vi "3D Single Mouse Movie.vi"() -> ()   [LabVIEW 2011]
uses:
  <vilib>/Native 3D Graph/xcontrol/3DPC_SurfacePlot.xctl
  <vilib>/Analysis/3filter.llb/Filter Passband Type.ctl
  <vilib>/Utility/file.llb/Write To Spreadsheet File (string).vi
  <vilib>/Analysis/1siggen.llb/Ramp Pattern by Samples.vi
  <vilib>/measure/mascope.llb/Transition Measurements 1 chan.vi
  <vilib>/Utility/file.llb/Write To Spreadsheet File (DBL).vi
  <vilib>/gmath/statdist.llb/Wilcoxon Signed-Rank Test (mean).vi
  <vilib>/vision/NI_Vision_Development_Module.lvlib
  <vilib>/Analysis/NI_AALBase.lvlib
  <vilib>/ptbypt/NI_PtbyPt.lvlib
  <vilib>/gmath/NI_Gmath.lvlib
  <vilib>/Analysis/NI_AALPro.lvlib
  <vilib>/Analysis/NI_AAL_Geometry.lvlib
  <vilib>/measure/NI_MAPro.lvlib
panel:
  out "Particle Measurements (Pixels)":dbl[][](array[numeric]) format="%.2f"
  in  "Selection Values":T2(array[cluster]) {"Measurement Parameter" items=["Center of Mass X", "Center of Mass Y", "First Pixel X", "First Pixel Y", "Bounding Rect Left", "Bounding Rect Top", "Bounding Rect Right", "Bounding Rect Bottom", "Max Feret Diameter Start X", "Max Feret Diameter Start Y", "Max Feret Diameter End X", "Max Feret Diameter End Y", "Max Horiz. Segment Length Left", "Max Horiz. Segment Length Right", "Max Horiz. Segment Length Row", "-", "Bounding Rect Width", "Bounding Rect Height", "Bounding Rect Diagonal", "Perimeter", "Convex Hull Perimeter", "Holes' Perimeter", "Max Feret Diameter", "Equivalent Ellipse Major Axis", "Equivalent Ellipse Minor Axis", "Equivalent Ellipse Minor Axis (Feret)", "Equivalent Rect Long Side", "Equivalent Rect Short Side", "Equivalent Rect Diagonal", "Equivalent Rect Short Side (Feret)", "Average Horiz. Segment Length", "Average Vert. Segment Length", "Hydraulic Radius", "Waddel Disk Diameter", "-", "Area", "Holes' Area", "Particle & Holes' Area", "Convex Hull Area", "Image Area", "-", "Number of Holes", "Number of Horiz. Segments", "Number of Vert. Segments", "-", "Orientation", "Max Feret Diameter Orientation", "-", "% Area/Image Area", "% Area/(Particle & Holes' Area)", "Ratio of Equivalent Ellipse Axes", "Ratio of Equivalent Rect Sides", "-", "Elongation Factor", "Compactness Factor", "Heywood Circularity Factor", "Type Factor", "-", "Sum X", "Sum Y", "Sum XX", "Sum XY", "Sum YY", "Sum XXX", "Sum XXY", "Sum XYY", "Sum YYY", "-", "Moment of Inertia XX", "Moment of Inertia XY", "Moment of Inertia YY", "Moment of Inertia XXX", "Moment of Inertia XXY", "Moment of Inertia XYY", "Moment of Inertia YYY", "Norm. Moment of Inertia XX", "Norm. Moment of Inertia XY", "Norm. Moment of Inertia YY", "Norm. Moment of Inertia XXX", "Norm. Moment of Inertia XXY", "Norm. Moment of Inertia XYY", "Norm. Moment of Inertia YYY", "Hu Moment 1", "Hu Moment 2", "Hu Moment 3", "Hu Moment 4", "Hu Moment 5", "Hu Moment 6", "Hu Moment 7"]; "Range Lower Value" format="%.2f"; "Range Upper Value" format="%.2f"}
  out "3D Graph":refnum<class "Base Datatype.lvclass">[](xcontrol)
  out "Spine Area v Max Height, 1 second history":T3(graph)
  in  "Image Folder":path=path "C:/Users/Behavior Room/Desktop/Recordings/Mouse 3"
  in  "Recording File":path=path "C:/Users/Behavior Room/Dropbox/Science/Datta lab/Kinect Mouse/Analysis/Blah.csv"
  in  "low cutoff freq: fl":dbl=0.125 format="%0.3f"
  out "Velocity":dbl(slide) scale=0.0..10.0
  in  "Flip?":bool
  in  "Butt Position":i32=10
  in  "threshold":dbl=100.0
  in  "Width of Band to \nCalculate Average Contour":i32=10
  out "Height":dbl(graph)
  out "Heat Map":T4(plugin-control)
  in  "Kernel Size":i32=11
  out "Right":bool
  out "Left":bool
  out "Is Significant":bool
  out "Half-Image Variance":T5(graph)
  out "Cross-Sectional Contour":cluster{"Y Max":i16[], "Ramp Pattern":dbl[]}(graph)
  out "Spine Contour":i16[][](graph) caption="X"
  in  "3D options":T6={"alpha"=15.0, "beta"=31.0, "border"=20, "background"=85, "plane"=2} {"beta" min=15 max=45 format="%.2f"; "alpha" min=15 max=45 format="%.2f"}
  in  "Direction (NW)":T7(ring)
  in  "Maximum height":i32=20
  in  "Size reduction":i32=1
  out "3D Experiment Area View":T4(plugin-control)
  out "Just Mouse":T4(plugin-control)
  out "Image #":i32
  out "Image":T4(plugin-control)
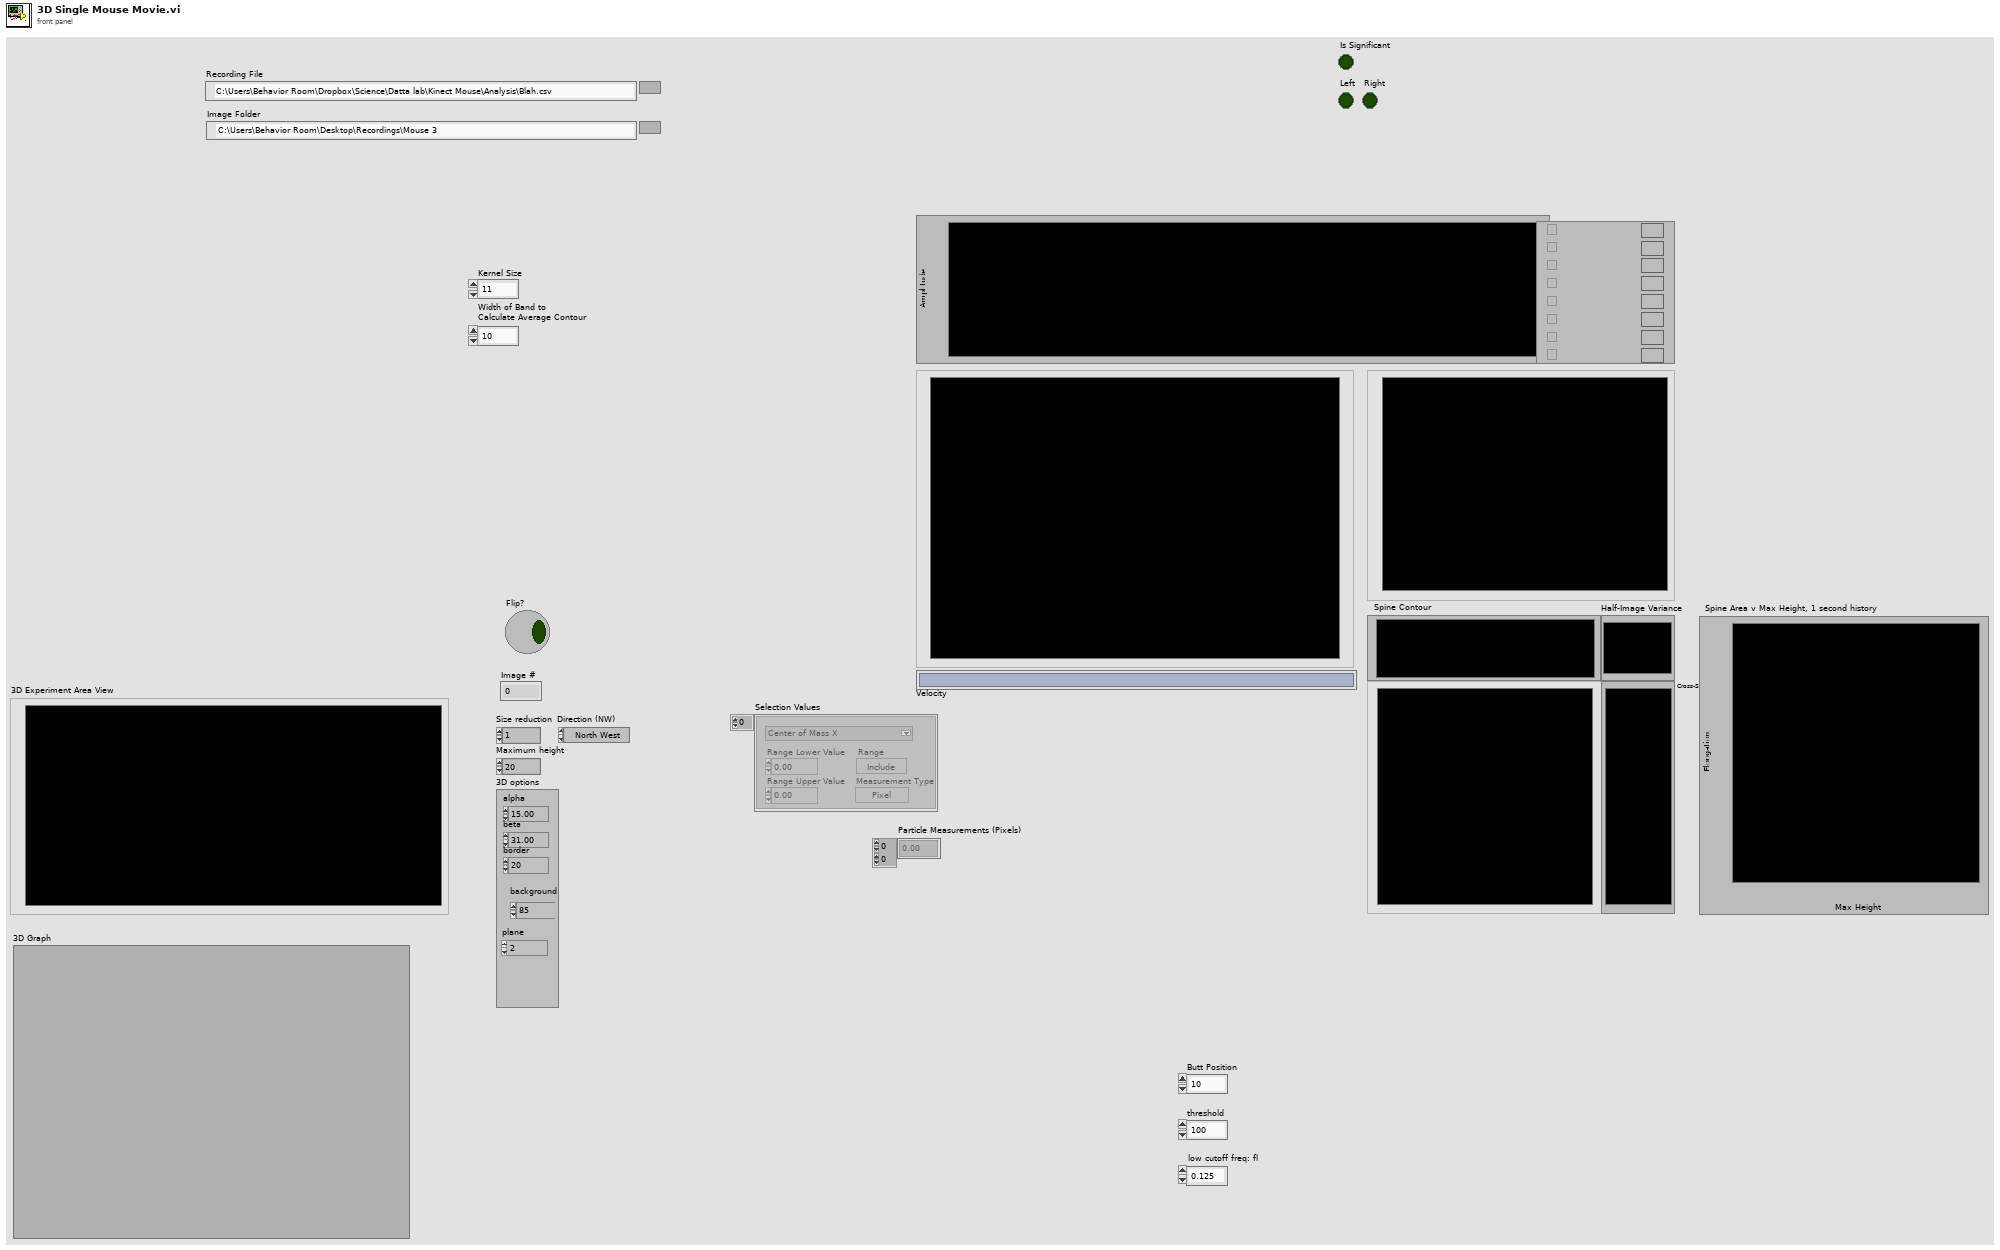
[diagram p1: front panel]
types:
  T1 = typedef "Particle Parameters" = i32
  T2 = cluster{"Measurement Parameter":T1, "Range Lower Value":dbl, "Range Upper Value":dbl, "Range":bool, "Measurement Type":bool}[]
  T3 = cluster{"Current Queue":dbl[], "Current Queue":dbl[]}
  T4 = typedef "IMAQ Image.ctl" = refnum<image>
  T5 = cluster{"standard deviation":dbl, "standard deviation":dbl}
  T6 = cluster{"alpha":sgl, "beta":sgl, "border":i32, "background":i32, "plane":i32}
  T7 = enum32{"North West", "South West", "South East", "North East"}
  T8 = typedef "Image Type" = u32
  T9 = typedef "NI_AALBase.lvlib/Filter Passband Type.ctl" = enum32{"Lowpass", "Highpass", "Bandpass", "Bandstop"}
  T10 = cluster{"Area":dbl, "Number of Holes":dbl, "Bounding Rect":cluster{"Left":dbl, "Top":dbl, "Right":dbl, "Bottom":dbl}, "Center of Mass":cluster{"X":dbl, "Y":dbl}, "Orientation":dbl, "Dimensions":cluster{"Width":dbl, "Height":dbl}}[]
  T11 = cluster{"high ref level":dbl, "mid ref level":dbl, "low ref level":dbl, "ref units":u16}
  T12 = cluster{"Area":dbl, "Number of Holes":dbl, "Bounding Rect":cluster{"Left":dbl, "Top":dbl, "Right":dbl, "Bottom":dbl}, "Center of Mass":cluster{"X":dbl, "Y":dbl}, "Orientation":dbl, "Dimensions":cluster{"Width":dbl, "Height":dbl}}
  T13 = cluster{"start time":dbl, "end time":dbl, "ref levels":cluster{"high ref level":dbl, "mid ref level":dbl, "low ref level":dbl, "ref units":u16}}
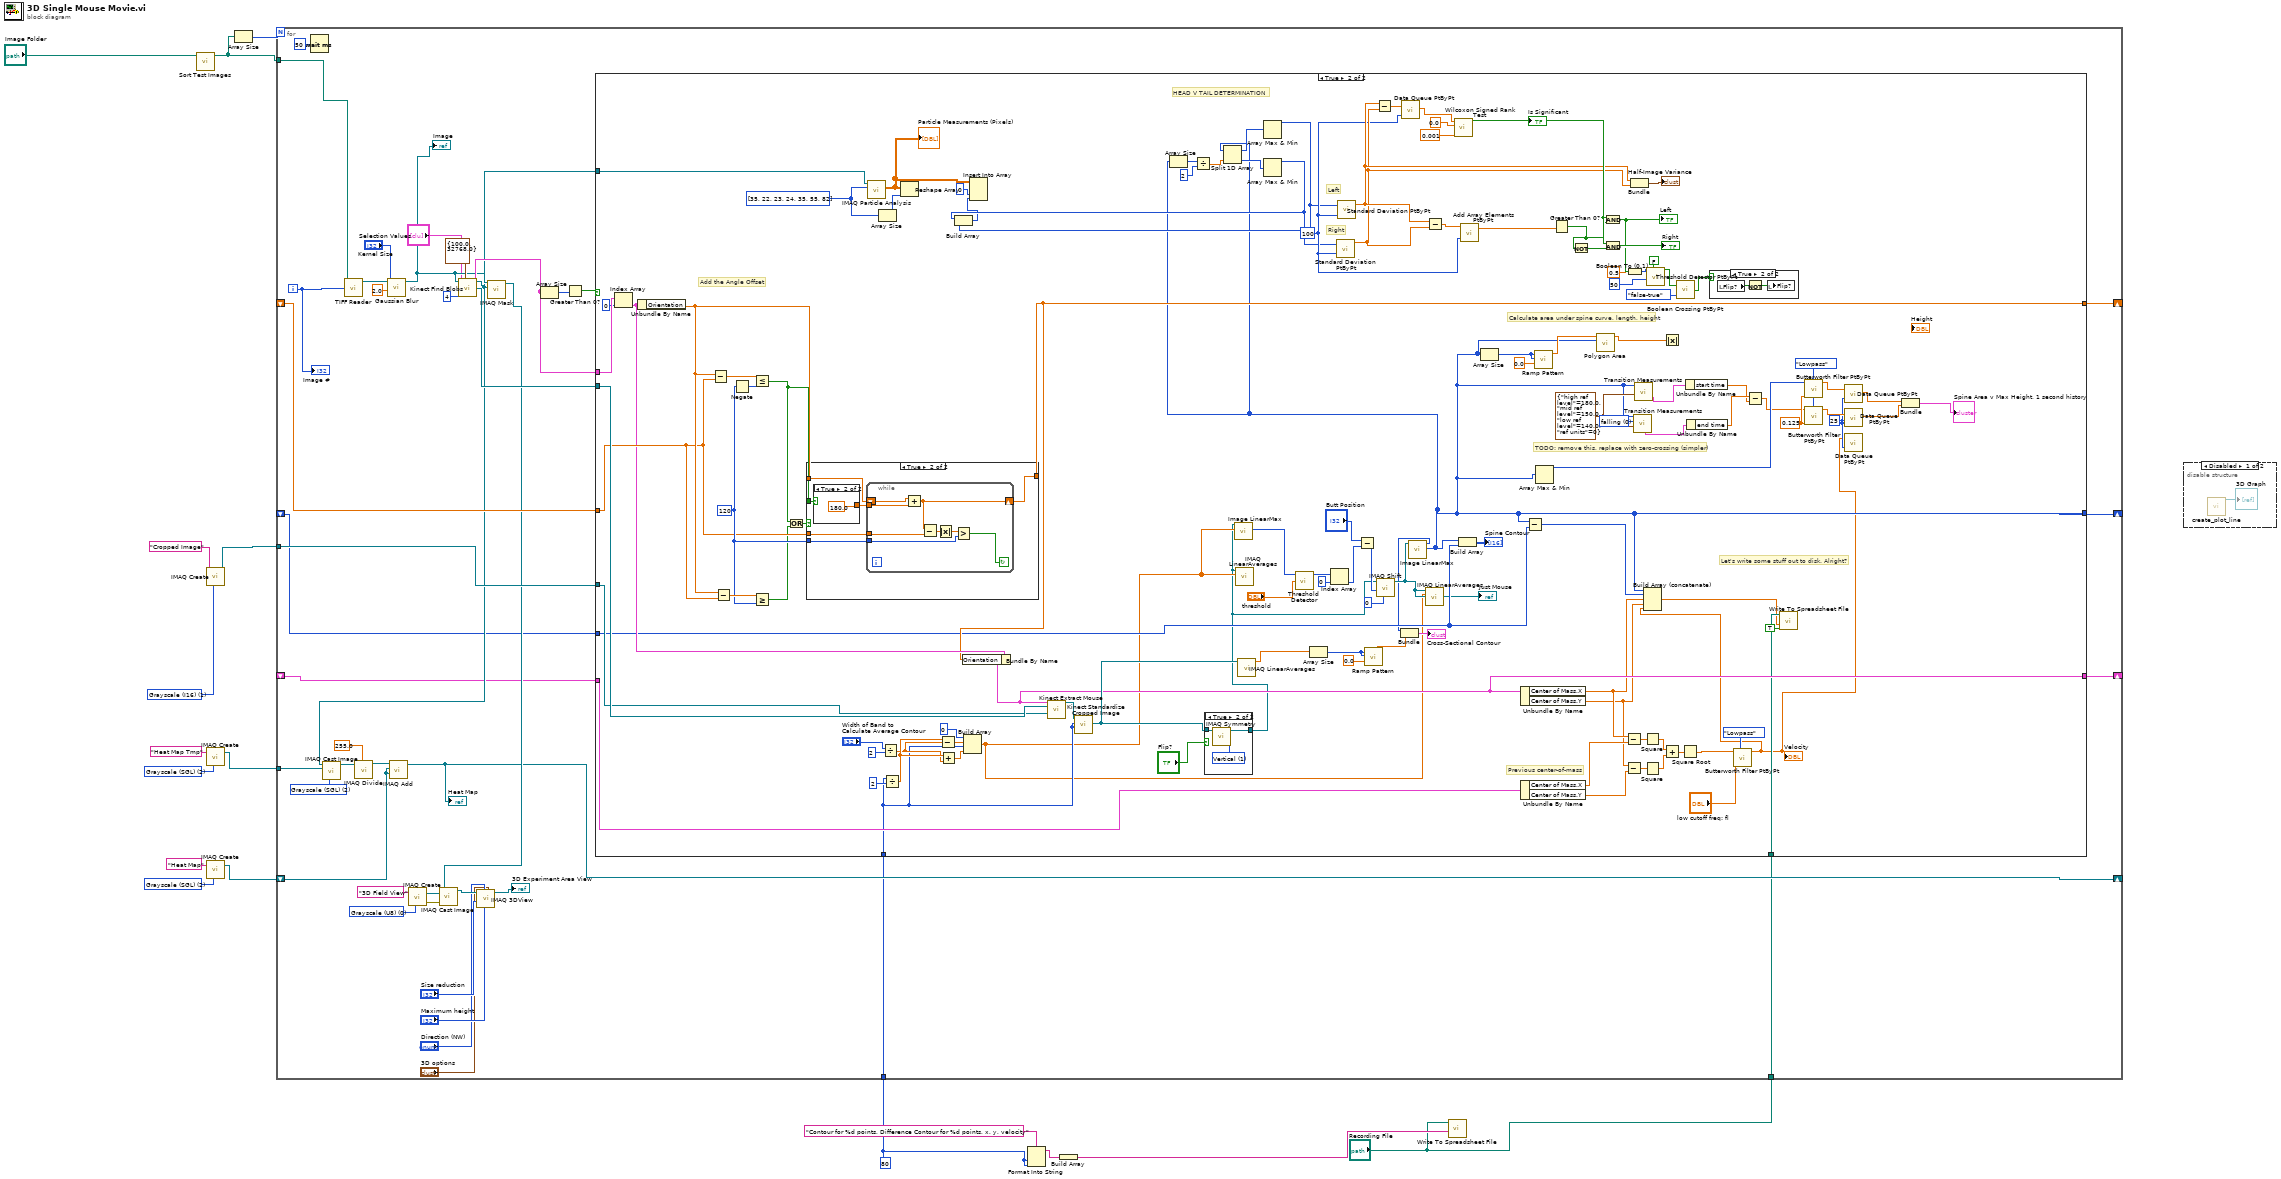
[diagram p0: block diagram]
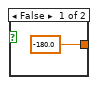
[diagram p6: hidden frame]
diagram:
  w4 = 80 ("Width")
  w7 = T8 2 items=["Grayscale (U8)", "Grayscale (I16)", "Grayscale (SGL)", "Complex (CSG)", "RGB (U32)", "HSL (U32)", "RGB (U64)", "Grayscale (U16)"] ("Image Type")
  w11 = T8 2 items=["Grayscale (U8)", "Grayscale (I16)", "Grayscale (SGL)", "Complex (CSG)", "RGB (U32)", "HSL (U32)", "RGB (U64)", "Grayscale (U16)"] ("Image Type")
  w14 = T8 1 items=["Grayscale (U8)", "Grayscale (I16)", "Grayscale (SGL)", "Complex (CSG)", "RGB (U32)", "HSL (U32)", "RGB (U64)", "Grayscale (U16)"] ("Image Type")
  n1 = call "Sort Test Images.vi"("path"="Image Folder") -> ("Array"=w16:path[])  [unwired: 10 in]
  n2 = call "IMAQ Create"("Image Name"="Cropped Image", "Image Type"=w14) -> ("New Image"=w13:T4)  [unwired: 3 in, 1 out]
  n3 = call "IMAQ Create"("Image Name"="Heat Map Tmp", "Image Type"=w7) -> ("New Image"=w6:T4)  [unwired: 3 in, 1 out]
  n4 = call "IMAQ Create"("Image Name"="Heat Map", "Image Type"=w11) -> ("New Image"=w9:T4)  [unwired: 3 in, 1 out]
  n5 = Array Size(array=w16) -> (size(s)=w17:i32)
  n6 = for {
    N: w17 -> [_]
    tunnel: w16 -> [w59]
    tunnel: w13 -> [w53]
    shift-right: [w51] -> _
    shift-left: _ -> [w50]
    shift-right: [w31] -> _
    shift-left: w9 -> [w32]
    tunnel: w6 -> [w28]
    shift-right: [w24] -> _
    shift-left: _ -> [w23]
    shift-right: [w22] -> _
    shift-left: _ -> [w21]
    tunnel: w4 -> [w20]
    tunnel: "Recording File" -> [w19]
    i -> [w58]
    w30 = T8 2 items=["Grayscale (U8)", "Grayscale (I16)", "Grayscale (SGL)", "Complex (CSG)", "RGB (U32)", "HSL (U32)", "RGB (U64)", "Grayscale (U16)"] ("Image Type")
    w47 = T8 0 items=["Grayscale (U8)", "Grayscale (I16)", "Grayscale (SGL)", "Complex (CSG)", "RGB (U32)", "HSL (U32)", "RGB (U64)", "Grayscale (U16)"] ("Image Type")
    n7 = Wait (ms)(milliseconds to wait=u32 50) -> ()  [unwired: 1 out]
    n8 = call "TIFF Reader.vi"("index"=w58, "Array"=w59) -> ("Image Out"=w36:T4)  [unwired: 9 in]
    n9 = call "Gaussian Blur.vi"("Standard Deviation"=2.0, "Kernel Size"="Kernel Size", "Image"=w36) -> ("Image Out"=w34:T4)  [unwired: 8 in]
    "Image" <- w34
    n10 = call "IMAQ Create"("Image Name"="3D Field View", "Image Type"=w47) -> ("New Image"=w45:T4, "error out"=w46:errorcluster)  [unwired: 3 in]
    n11 = call "Kinect Find Blobs.vi"("Image Src"=w34, "Range"=cluster{"Lower value":sgl, "Upper value":sgl} {"Lower value"=100.0, "Upper value"=32768.0}, "Selection Values"="Selection Values", "Number of Erosion"=4) -> ("Masked Image Out"=w25:T4, "Particle Reports (Pixels)"=w54:T10, "Src Image Out"=w52:T4)  [unwired: 8 in, 1 out]
    n12 = call "IMAQ Cast Image"("Image Type"=w30, "Image Dst"=w28, "Image Src"=w25) -> ("Image Dst Out"=w29:T4)  [unwired: 7 in, 1 out]
    n13 = call "IMAQ Divide"("Image Src A"=w29, "Constant"=sgl 255.0) -> ("Image Dst Out"=w26:T4)  [unwired: 5 in, 1 out]
    n14 = call "IMAQ Add"("Image Src A"=w26, "Image Dst"=w32, "Image Src B"=w32) -> ("Image Dst Out"=w31:T4)  [unwired: 4 in, 1 out]
    "Heat Map" <- w31
    n15 = call "IMAQ Mask"("Image Mask"=w25, "Image Src"=w34) -> ("Image Dst Out"=w38:T4)  [unwired: 3 in, 1 out]
    n16 = call "IMAQ Cast Image"("error in (no error)"=w46, "Image Dst"=w45, "Image Src"=w38) -> ("Image Dst Out"=w44:T4)  [unwired: 7 in, 1 out]
    n17 = call "IMAQ 3DView"("3D options"="3D options", "Maximum height"="Maximum height", "Direction (NW)"="Direction (NW)", "Size reduction"="Size reduction", "Image Src"=w44) -> ("Image Dst Out"=→"3D Experiment Area View":T4)  [unwired: 5 in, 1 out]
    n18 = Array Size(array=w54) -> (size(s)=w56:i32)
    n19 = Greater Than 0?(x=w56) -> (x > 0?=w55:bool)
    n20 = case shown="True" w55 {
      tunnel: w54 -> [_ w183]
      tunnel: w52 -> [_ w181]
      tunnel: w53 -> [_ w180]
      tunnel: [w62 w129] -> w51
      tunnel: w50 -> [w62 w134]
      tunnel: w25 -> [_ w147]
      tunnel: [w61 w74] -> w24
      tunnel: w23 -> [w61 w111]
      tunnel: [w60 w108] -> w22
      tunnel: w21 -> [w60 w107]
      tunnel: w20 -> [_ w94]
      tunnel: w19 -> [_ w93]
      frame False {
      }
      frame True {
        w71 = 0.125 ("low cutoff freq: fl")
        w72 = Filter_Passband_Type."Lowpass" ("filter type")
        w66 = 25 ("sample length")
        w78 = u16 0 items=["falling", "rising"] ("polarity (rising)")
        w79 = T11 {"high ref level"=180.0, "mid ref level"=150.0, "low ref level"=140.0, "ref units"=0} ("reference levels")
        w136 = 120
        w146 = T1[] [35, 22, 23, 24, 35, 55, 82] items=["Center of Mass X", "Center of Mass Y", "First Pixel X", "First Pixel Y", "Bounding Rect Left", "Bounding Rect Top", "Bounding Rect Right", "Bounding Rect Bottom", "Max Feret Diameter Start X", "Max Feret Diameter Start Y", "Max Feret Diameter End X", "Max Feret Diameter End Y", "Max Horiz. Segment Length Left", "Max Horiz. Segment Length Right", "Max Horiz. Segment Length Row", "-", "Bounding Rect Width", "Bounding Rect Height", "Bounding Rect Diagonal", "Perimeter", "Convex Hull Perimeter", "Holes' Perimeter", "Max Feret Diameter", "Equivalent Ellipse Major Axis", "Equivalent Ellipse Minor Axis", "Equivalent Ellipse Minor Axis (Feret)", "Equivalent Rect Long Side", "Equivalent Rect Short Side", "Equivalent Rect Diagonal", "Equivalent Rect Short Side (Feret)", "Average Horiz. Segment Length", "Average Vert. Segment Length", "Hydraulic Radius", "Waddel Disk Diameter", "-", "Area", "Holes' Area", "Particle & Holes' Area", "Convex Hull Area", "Image Area", "-", "Number of Holes", "Number of Horiz. Segments", "Number of Vert. Segments", "-", "Orientation", "Max Feret Diameter Orientation", "-", "% Area/Image Area", "% Area/(Particle & Holes' Area)", "Ratio of Equivalent Ellipse Axes", "Ratio of Equivalent Rect Sides", "-", "Elongation Factor", "Compactness Factor", "Heywood Circularity Factor", "Type Factor", "-", "Sum X", "Sum Y", "Sum XX", "Sum XY", "Sum YY", "Sum XXX", "Sum XXY", "Sum XYY", "Sum YYY", "-", "Moment of Inertia XX", "Moment of Inertia XY", "Moment of Inertia YY", "Moment of Inertia XXX", "Moment of Inertia XXY", "Moment of Inertia XYY", "Moment of Inertia YYY", "Norm. Moment of Inertia XX", "Norm. Moment of Inertia XY", "Norm. Moment of Inertia YY", "Norm. Moment of Inertia XXX", "Norm. Moment of Inertia XXY", "Norm. Moment of Inertia XYY", "Norm. Moment of Inertia YYY", "Hu Moment 1", "Hu Moment 2", "Hu Moment 3", "Hu Moment 4", "Hu Moment 5", "Hu Moment 6", "Hu Moment 7"] ("Pixel Measurements")
        w150 = 100 ("sample length")
        # "TODO: remove this, replace with zero-crossing (simpler)"
        # "Calculate area under spine curve, length, height"
        # "HEAD V TAIL DETERMINATION"
        # "Previous center-of-mass"
        # "Let's write some stuff out to disk. Alright?"
        # "Right"
        # "Left"
        # "Add the Angle Offset"
        n21 = Index Array(array=w183, index=0) -> (element=w130:T12)
        n22 = Unbundle By Name(w130) -> ("Orientation"=w135:dbl)
        n23 = Subtract(x=w135, y=w134) -> (x-y=w139:dbl)
        n24 = Subtract(x=w135, y=w134) -> (x-y=w137:dbl)
        n25 = Negate(x=w136) -> (-x=w138:i32)
        n26 = Less Or Equal?(x=w139, y=w138) -> (x <= y?=w131:bool)
        n27 = Greater Or Equal?(x=w137, y=w136) -> (x >= y?=w133:bool)
        n28 = Or(x=w131, y=w133) -> (x .or. y?=w132:bool)
        n29 = case shown="True" w132 {
          tunnel: [w186 w192] -> w129
          tunnel: w136 -> [_ w191]
          tunnel: w135 -> [w186 w190]
          tunnel: w134 -> [_ w189]
          tunnel: w131 -> [_ w188]
          frame False {
          }
          frame True {
            n30 = case shown="True" w188 {
              tunnel: [-180.0 ("y") 180.0 ("y")] -> w187
              frame False {
              }
              frame True {
              }
            }
            n31 = while {
              tunnel: w189 -> [w200]
              tunnel: w191 -> [w197]
              tunnel: w187 -> [w195]
              shift-right: [w201] -> w192
              shift-left: w190 -> [w202]
              stop <- w196 continue-if-true
              n32 = Add(x=w202, y=w195) -> (x+y=w201:dbl)
              n33 = Subtract(x=w201, y=w200) -> (x-y=w199:dbl)
              n34 = Absolute Value(x=w199) -> (abs(x)=w198:dbl)
              n35 = Greater?(x=w198, y=w197) -> (0:w196:bool)
            }
          }
        }
        n36 = call "IMAQ Particle Analysis"("Pixel Measurements"=w146, "Image"=w147) -> ("Particle Measurements (Pixels)"=w144:dbl[][])  [unwired: 4 in, 5 out]
        "Particle Measurements (Pixels)" <- w144
        n37 = Array Size(array=w146) -> (size(s)=w145:i32)
        n38 = Divide(x="Width of Band to \nCalculate Average Contour", y=2) -> (x/y=w167:dbl)
        n39 = Divide(x=w94, y=2) -> (x/y=w168:dbl)
        n40 = Reshape Array(w144, w145) -> ()  [unwired: 1 out]
        n41 = Subtract(x=w168, y=w167) -> (x-y=w170:dbl)
        n42 = Add(x=w168, y=w167) -> (x+y=w169:dbl)
        n43 = Bundle By Name(cluster=w130, "Orientation"=w129) -> (w108:T12)
        n44 = Build Array(0 ("element"), w170, w94, w169) -> (w87:dbl[])
        n45 = call "Kinect Extract Mouse.vi"("Particle Report"=w108, "Image Src"=w181, "Image Dst"=w180) -> ("Cropped Image Out"=w175:T4)  [unwired: 11 in, 1 out]
        n46 = call "Kinect Standardize Cropped Image.vi"("Height"=w94, "Width"=w94, "Image"=w175) -> ("Image Dst Out"=w149:T4)  [unwired: 7 in, 1 out]
        n47 = case shown="True" "Flip?" {
          tunnel: [w203 w206] -> w86
          tunnel: w149 -> [w203 w205]
          frame False {
          }
          frame True {
            w204 = u32 1 items=["Horizontal", "Vertical", "Central", "1st Diagonal", "2nd Diagonal"] ("Type of Symmetry")
            n48 = call "IMAQ Symmetry"("Type of Symmetry"=w204, "Image Src"=w205) -> ("Image Dst Out"=w206:T4)  [unwired: 3 in, 1 out]
          }
        }
        n49 = call "Image LinearMax.vi"("Optional Rectangle"=w87, "Image Src"=w86) -> ("X Max"=w88:i16[])  [unwired: 7 in, 2 out]
        n50 = call "IMAQ LinearAverages"("Optional Rectangle"=w87, "Image Src"=w86) -> ()  [unwired: 5 in, 5 out]
        n51 = call "IMAQ LinearAverages"("Image Src"=w149) -> ("Y Axis Averages"=w148:sgl[])  [unwired: 6 in, 4 out]
        n52 = call <vilib>:"Threshold Detector.vi"("threshold"="threshold", "X"=w88) -> ("Indices"=w128:i32[])  [unwired: 1 in, 2 out]
        n53 = Array Size(array=w148) -> (size(s)=w177:i32)
        n54 = Index Array(array=w128, index=0) -> (element=w125:i32)
        n55 = Subtract(x="Butt Position", y=w125) -> (x-y=w124:i32)
        n56 = call-poly <vilib>:"Ramp Pattern.vi"("start"=0.0, "end"=w177, "samples"=w177) -> ("Ramp Pattern"=w178:dbl[])  [unwired: 7 in, 1 out]
        n57 = call "IMAQ Shift"("YOffset"=0, "XOffset"=w124, "Image Src"=w86) -> ("Image Dst Out"=w90:T4)  [unwired: 7 in, 1 out]
        "Just Mouse" <- w90
        n58 = call "Image LinearMax.vi"("Image Src"=w90) -> ("X Max"=w74:i16[], "Y Max"=w89:i16[])  [unwired: 8 in, 1 out]
        n59 = Array Size(array=w74) -> (size(s)=w163:i32)
        n60 = Divide(x=w163, y=2) -> (x/y=w162:dbl)
        n61 = Split 1D Array(array=w74, index=w162) -> (first subarray=w166:i16[], second subarray=w165:i16[])
        n62 = Array Max & Min(array=w166) -> (max value=w142:i16)  [unwired: 3 out]
        n63 = Array Max & Min(array=w165) -> (max value=w143:i16)  [unwired: 3 out]
        n64 = Build Array(w143, w142) -> (w141:i16[])
        n65 = Insert Into Array(array=w144, index (col)=0 ("index (row)"), new element=w141) -> ()  [unwired: 1 in, 1 out]
        n66 = call <vilib>:"Standard Deviation PtByPt.vi"("x"=w143, "sample length"=w150) -> ("standard deviation"=w153:dbl)  [unwired: 1 in, 2 out]
        n67 = call <vilib>:"Standard Deviation PtByPt.vi"("x"=w142, "sample length"=w150) -> ("standard deviation"=w154:dbl)  [unwired: 1 in, 2 out]
        n68 = Subtract(x=w154, y=w153) -> (x-y=w157:dbl)
        n69 = Bundle("Y Max"=w89, "Ramp Pattern"=w178) -> (→"Cross-Sectional Contour":cluster{"Y Max":i16[], "Ramp Pattern":dbl[]})  [unwired: 1 in]
        n70 = call <vilib>:"Data Queue PtByPt.vi"("input data point"=w157, "sample length"=w150) -> ("Current Queue"=w160:dbl[])  [unwired: 1 in, 4 out]
        n71 = call "IMAQ LinearAverages"("Optional Rectangle"=w87, "Image Src"=w90) -> ()  [unwired: 5 in, 5 out]
        n72 = Subtract(x=w154, y=w153) -> (x-y=w152:dbl)
        n73 = call-poly <vilib>:"Wilcoxon Signed Rank Test.vi"("significance level"=0.001, "mean"=0.0, "sample set"=w160) -> ("reject null hypothesis"=w155:bool)  [unwired: 6 in, 2 out]
        "Is Significant" <- w155
        n74 = Build Array(w74, w111) -> (→"Spine Contour":i16[][])
        n75 = call <vilib>:"Add Array Elements PtByPt.vi"("sample length"=w150, "input data point"=w152) -> ("sum"=w151:dbl)  [unwired: 2 in, 1 out]
        n76 = Array Size(array=w74) -> (size(s)=w85:i32)
        n77 = Unbundle By Name(w108) -> ("Center of Mass.X"=w106:dbl, "Center of Mass.Y"=w104:dbl)
        n78 = Unbundle By Name(w107) -> ("Center of Mass.X"=w105:dbl, "Center of Mass.Y"=w103:dbl)
        n79 = Subtract(x=w74, y=w111) -> (x-y=w109:i16[])
        n80 = call-poly <vilib>:"Ramp Pattern.vi"("start"=0.0, "end"=w85, "samples"=w85) -> ("Ramp Pattern"=w83:dbl[])  [unwired: 7 in, 1 out]
        n81 = Array Max & Min(array=w74) -> (max value=w68:i16)  [unwired: 3 out]
        n82 = Greater Than 0?(x=w151) -> (x > 0?=w120:bool)
        n83 = Not(x=w120) -> (.not. x?=w156:bool)
        n84 = call <vilib>:"Polygon Area.vi"("Y"=w74, "X"=w83) -> ("signed area"=w82:dbl)  [unwired: 8 in, 1 out]
        n85 = And(x=w155, y=w120) -> (x .and. y?=w118:bool)
        "Left" <- w118
        n86 = And(x=w155, y=w156) -> (x .and. y?=→"Right":bool)
        n87 = Subtract(x=w106, y=w105) -> (x-y=w102:dbl)
        n88 = Subtract(x=w104, y=w103) -> (x-y=w101:dbl)
        n89 = Boolean To (0,1)(Boolean=w118) -> (0, 1=w119:i16)
        n90 = Bundle("standard deviation"=w154, "standard deviation"=w153) -> (→"Half-Image Variance":T5)  [unwired: 1 in]
        n91 = call-poly <vilib>:"Transition Measurements.vi"("reference levels"=w79, "polarity (rising)"=w78, "signal in"=w74) -> ("measurement info"=w77:T13)  [unwired: 3 in, 5 out]
        n92 = call-poly <vilib>:"Transition Measurements.vi"("reference levels"=w79, "signal in"=w74) -> ("measurement info"=w80:T13)  [unwired: 4 in, 5 out]
        n93 = Square(x=w102) -> (x^2=w100:dbl)
        n94 = Square(x=w101) -> (x^2=w99:dbl)
        n95 = call <vilib>:"Threshold Detector PtByPt.vi"("initialize"=FALSE, "width"=50, "threshold"=0.5, "x"=w119) -> ("detected"=w116:bool)  [unwired: 5 in, 2 out]
        n96 = Absolute Value(x=w82) -> ()  [unwired: 1 out]
        n97 = Add(x=w100, y=w99) -> (x+y=w98:dbl)
        n98 = call <vilib>:"Boolean Crossing PtByPt.vi"("direction"=enum16{"either", "false-true", "true-false"}."false-true", "input"=w116) -> ("crossing"=w115:bool)  [unwired: 1 in]
        n99 = Square Root(x=w98) -> (sqrt(x)=w97:dbl)
        n100 = Unbundle By Name(w80) -> ("start time"=w75:dbl)
        n101 = Unbundle By Name(w77) -> ("end time"=w76:dbl)
        n102 = case shown="True" w115 {
          frame False {
          }
          frame True {
            n103 = local read "Flip?"() -> (w185:bool)
            n104 = Not(x=w185) -> (.not. x?=w184:bool)
            n105 = local write "Flip?"(w184) -> ()
          }
        }
        n106 = call <vilib>:"Butterworth Filter PtByPt.vi"("filter type"=Filter_Passband_Type."Lowpass", "low cutoff freq: fl"="low cutoff freq: fl", "x"=w97) -> ("Filtered x"=w65:dbl)  [unwired: 6 in, 1 out]
        "Velocity" <- w65
        n107 = Build Array (concatenate)(w74, w109, w106, w104, w65) -> (w91:dbl[])
        n108 = Subtract(x=w76, y=w75) -> (x-y=w67:dbl)
        n109 = call-poly <vilib>:"Write To Spreadsheet File.vi"("append to file? (new file:F)"=TRUE, "1D data"=w91, "file path (dialog if empty)"=w93) -> ()  [unwired: 5 in, 1 out]
        n110 = call <vilib>:"Butterworth Filter PtByPt.vi"("filter type"=w72, "low cutoff freq: fl"=w71, "x"=w68) -> ("Filtered x"=w69:dbl)  [unwired: 6 in, 1 out]
        n111 = call <vilib>:"Butterworth Filter PtByPt.vi"("filter type"=w72, "low cutoff freq: fl"=w71, "x"=w67) -> ("Filtered x"=w70:dbl)  [unwired: 6 in, 1 out]
        n112 = call <vilib>:"Data Queue PtByPt.vi"("input data point"=w69, "sample length"=w66) -> ("Current Queue"=w63:dbl[])  [unwired: 1 in, 4 out]
        n113 = call <vilib>:"Data Queue PtByPt.vi"("input data point"=w70, "sample length"=w66) -> ("Current Queue"=w64:dbl[])  [unwired: 1 in, 4 out]
        n114 = call <vilib>:"Data Queue PtByPt.vi"("input data point"=w65, "sample length"=w66) -> ()  [unwired: 1 in, 5 out]
        n115 = Bundle("Current Queue"=w63, "Current Queue"=w64) -> (→"Spine Area v Max Height, 1 second history":T3)  [unwired: 1 in]
      }
    }
    "Image #" <- w58
  }
  n116 = Format Into String(format string="Contour for %d points, Difference Contour for %d points, x, y, velocity", w4, w4) -> (resulting string=w3:string)  [unwired: 2 in, 1 out]
  n117 = Build Array(w3) -> (w2:string[])
  n118 = call-poly <vilib>:"Write To Spreadsheet File.vi"("1D data"=w2, "file path (dialog if empty)"="Recording File") -> ()  [unwired: 6 in, 1 out]
  n119 = disable-structure shown="Disabled" {
    frame Disabled {
      n120 = call <vilib>:"create_plot_line.vi"() -> ("plots out"=→"3D Graph":refnum<class "Base Datatype.lvclass">[])  [unwired: 5 in, 6 out]
    }
    frame Enabled {
    }
  }
